vi "GetPaths.vi"(5 "error in (no error)":errorcluster) -> (14 "Root folder":path, 15 "Image folder":path, 16 "Image URL":string, 19 "error out":errorcluster)   [LabVIEW 2014, in "FrontPanelPublisher.lvlib" / "FrontPanelManager.lvclass"]
uses:
  FrontPanelManager.lvclass
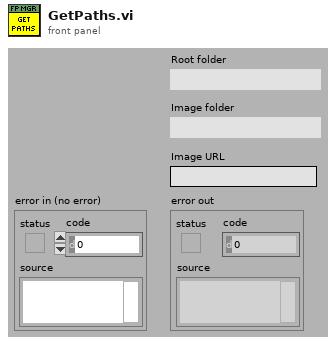
[diagram p1: front panel]
types:
  T1 = typedef "FrontPanelPublisher.lvlib/FrontPanelManager.lvclass/ObjectAttributes.ctl" = cluster{"WebFrontPanels":refnum<class "WebFrontPanel.lvclass">[], "WFP Names":string[], "Root folder":path, "Websocket Info":T2}
  T2 = typedef "FrontPanelPublisher.lvlib/FrontPanelManager.lvclass/WebsocketInfo.ctl" = cluster{"Hostname":string, "Port":u16}
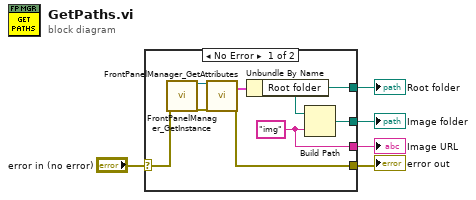
[diagram p0: block diagram]
diagram:
  n1 = case shown="No Error" "error in (no error)" {
    selector: "error in (no error)" -> [w10 w14]
    tunnel: [w12 w14] -> w4
    tunnel: [w8 _] -> w3
    tunnel: [w7 _] -> w2
    tunnel: [w6 _] -> w1
    frame No Error {
      w6 = "img" ("name or relative path")
      n2 = call "FrontPanelManager_GetInstance.vi"("error in (no error)"=w10) -> ("reference out"=w11:refnum<class "FrontPanelManager.lvclass">, "error out"=w9:errorcluster)  [unwired: 14 in, 3 out]
      n3 = call "FrontPanelManager_GetAttributes.vi"("reference in"=w11, "error in (no error)"=w9) -> ("Data"=w13:T1, "error out"=w12:errorcluster)  [unwired: 14 in, 2 out]
      n4 = Unbundle By Name(w13) -> ("Root folder"=w8:path)
      n5 = Build Path(base path=w8, name or relative path=w6) -> (appended path=w7:path)
    }
    frame Error {
    }
  }
  "error out" <- w4
  "Root folder" <- w3
  "Image folder" <- w2
  "Image URL" <- w1
